vi "OPCUA Refnum.vi"(3 "error in (no error)":errorcluster) -> (16 "OPC UA server refnum":refnum<k21>, 17 "error out":errorcluster)   [LabVIEW 2013, in "OPCUA(UtilityMode).lvlib"]
uses:
  OPCUA(UtilityMode).lvlib
  op(utility).ctl
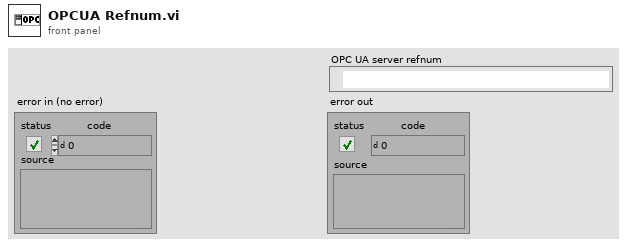
[diagram p1: front panel]
types:
  T1 = typedef "OPCUA(UtilityMode).lvlib/op(utility).ctl" = enum16{"Create Server", "Start Server", "Get Server Refnum", "Stop Server", "Close Server"}
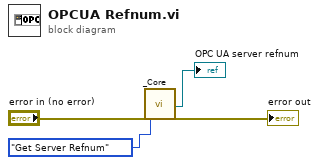
[diagram p0: block diagram]
diagram:
  n1 = call "_Core.vi"("error in (no error)"="error in (no error)", "Op"=op(utility)."Get Server Refnum") -> ("OPC UA server refnum"=→"OPC UA server refnum":refnum<k21>, "error out"=→"error out":errorcluster)  [unwired: 21 in, 3 out]
